vi "getYearAndDay.vi"() -> (0 "year":i32, 1 "Day of the year":dbl format="%#_13g")   [LabVIEW 2015]
panel:
  out "number of seconds between \nJanuary 1st 1904 and January 1st 2015":dbl format="%#_13g"
  out "number of seconds since the \nJanuary 1st 1904":dbl format="%#_13g"
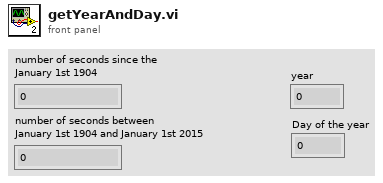
[diagram p1: front panel]
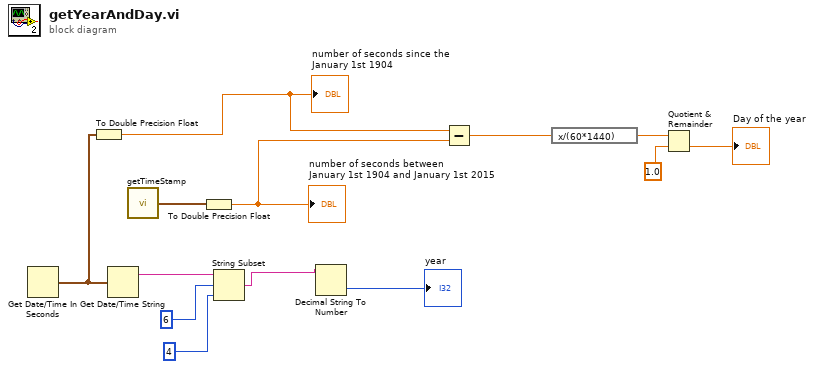
[diagram p0: block diagram]
diagram:
  (unwired) 6
  n1 = Get Date/Time In Seconds() -> (seconds since 1Jan1904=w8:timestamp)
  n2 = To Double Precision Float(number=w8) -> (double precision float=w6:dbl)
  "number of seconds since the \nJanuary 1st 1904" <- w6
  n3 = Get Date/Time String(seconds (now)=w8) -> (date string=w13:string)  [unwired: 2 in, 1 out]
  n4 = call "getTimeStamp.vi"() -> ("Time Stamp"=w7:timestamp)  [unwired: 2 in]
  n5 = To Double Precision Float(number=w7) -> (double precision float=w5:dbl)
  "number of seconds between \nJanuary 1st 1904 and January 1st 2015" <- w5
  n6 = String Subset(string=w13, offset (0)=6, length (rest)=4) -> (substring=w10:string)
  n7 = Decimal String To Number(string=w10) -> (number=→"year":i32)  [unwired: 2 in, 1 out]
  n8 = Subtract(x=w6, y=w5) -> (x-y=w4:dbl)
  n9 = expression code="x/(60*1440)"(w4) -> (w3:dbl)
  n10 = Quotient & Remainder(x=w3, y=1.0) -> (floor(x/y)=→"Day of the year":dbl)  [unwired: 1 out]
